vi "ClusterToArray_AssmeblyFeatures.vi"(11 "value":T1) -> (3 "Array":T2(array[cluster]))   [LabVIEW 2019]
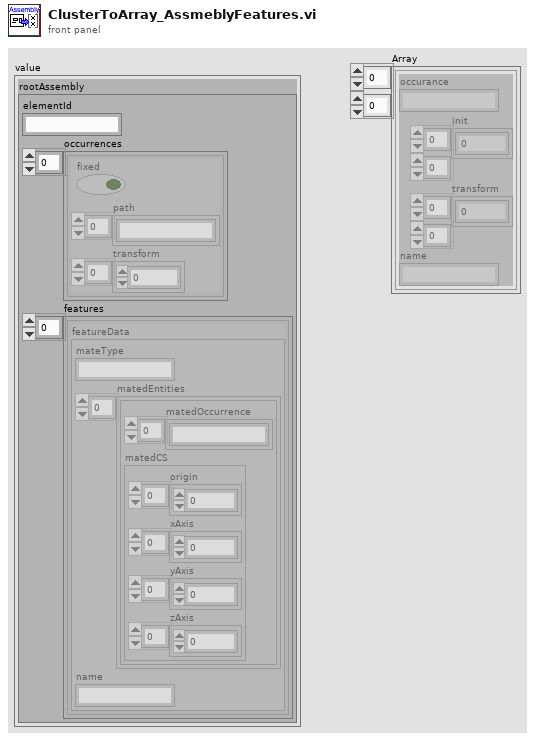
[diagram p1: front panel]
types:
  T1 = cluster{"rootAssembly":cluster{"elementId":string, "occurrences":cluster{"fixed":bool, "path":string[], "transform":dbl[]}[], "features":cluster{"featureData":cluster{"mateType":string, "matedEntities":cluster{"matedOccurrence":string[], "matedCS":cluster{"origin":dbl[], "xAxis":dbl[], "yAxis":dbl[], "zAxis":dbl[]}}[], "name":string}}[]}}
  T2 = cluster{"occurance":string, "init":dbl[][], "transform":dbl[][], "name":string}[][]
  T3 = cluster{"featureData":cluster{"mateType":string, "matedEntities":cluster{"matedOccurrence":string[], "matedCS":cluster{"origin":dbl[], "xAxis":dbl[], "yAxis":dbl[], "zAxis":dbl[]}}[], "name":string}}[]
  T4 = cluster{"fixed":bool, "path":string[], "transform":dbl[]}[]
  T5 = cluster{"occurance":string, "init":dbl[][], "transform":dbl[][], "name":string}
  T6 = cluster{"occurance":string, "init":dbl[][], "transform":dbl[][], "name":string}[]
  T7 = cluster{"matedOccurrence":string[], "matedCS":cluster{"origin":dbl[], "xAxis":dbl[], "yAxis":dbl[], "zAxis":dbl[]}}[]
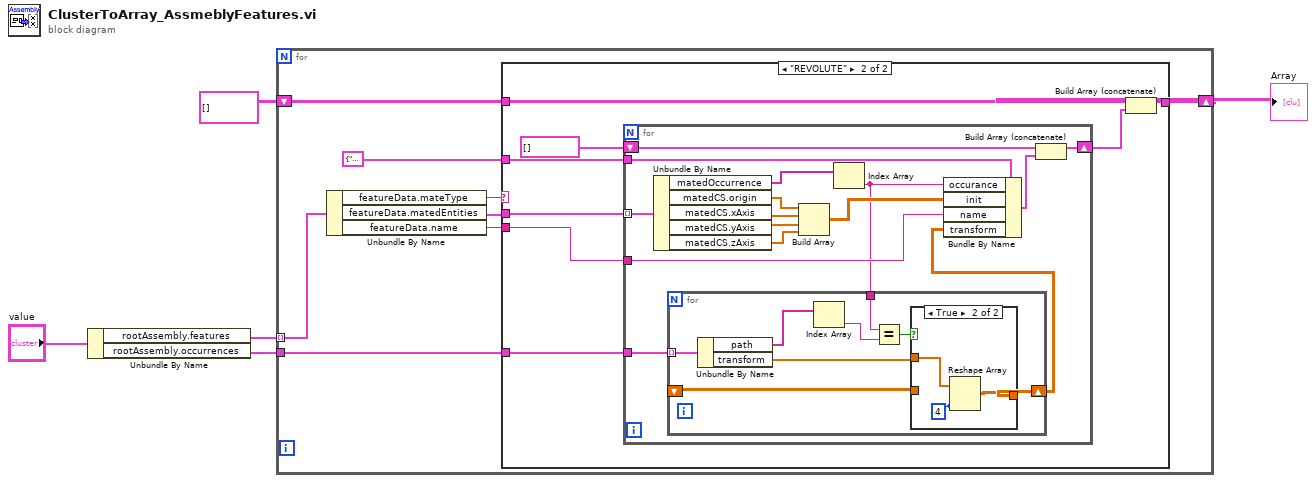
[diagram p0: block diagram]
diagram:
  n1 = Unbundle By Name("value") -> ("rootAssembly.features"=w2:T3, "rootAssembly.occurrences"=w5:T4)
  n2 = for {
    tunnel: w2 -> [w13] mode=indexing
    shift-right: [w7] -> w4
    shift-left: T2 [] -> [w8]
    tunnel: w5 -> [w6]
    n3 = Unbundle By Name(w13) -> ("featureData.mateType"=w12:string, "featureData.matedEntities"=w11:T7, "featureData.name"=w9:string)
    n4 = case shown="\"REVOLUTE\"" w12 {
      tunnel: w11 -> [_ w22]
      tunnel: T5 {"occurance"="", "init"=[], "transform"=[], "name"=""} -> [_ w21]
      tunnel: w9 -> [_ w15]
      tunnel: w8 -> [w14 w18]
      tunnel: [w14 w17] -> w7
      tunnel: w6 -> [_ w16]
      frame "False", Default {
      }
      frame "REVOLUTE" {
        n5 = for {
          tunnel: w22 -> [w37] mode=indexing
          tunnel: w21 -> [w36]
          shift-right: [w27] -> w19
          shift-left: T6 [] ("Array 2") -> [w26]
          tunnel: w15 -> [w29]
          tunnel: w16 -> [w25]
          n6 = Unbundle By Name(w37) -> ("matedOccurrence"=w35:string[], "matedCS.origin"=w34:dbl[], "matedCS.xAxis"=w33:dbl[], "matedCS.yAxis"=w32:dbl[], "matedCS.zAxis"=w31:dbl[])
          n7 = Build Array(w34, w33, w32, w31) -> (w30:dbl[][])
          n8 = Index Array(array=w35) -> (element=w24:string)  [unwired: 1 in]
          n9 = for {
            tunnel: w25 -> [w45] mode=indexing
            tunnel: w24 -> [w39]
            shift-right: [w41] -> w23
            shift-left: _ -> [w40]
            n10 = Unbundle By Name(w45) -> ("path"=w44:string[], "transform"=w42:dbl[])
            n11 = Index Array(array=w44) -> (element=w38:string)  [unwired: 1 in]
            n12 = Equal?(x=w39, y=w38) -> (x = y?=w43:bool)
            n13 = case shown="True" w43 {
              tunnel: w42 -> [_ w47]
              tunnel: [w46 w49] -> w41
              tunnel: w40 -> [w46 _]
              frame False {
              }
              frame True {
                w48 = 4 ("dimension size")
                n14 = Reshape Array(w47, w48, w48) -> (w49:dbl[][])
              }
            }
          }
          n15 = Bundle By Name(cluster=w36, "occurance"=w24, "init"=w30, "name"=w29, "transform"=w23) -> (w28:T5)
          n16 = Build Array (concatenate)(w26, w28) -> (w27:T6)
        }
        n17 = Build Array (concatenate)(w18, w19) -> (w17:T2)
      }
    }
  }
  "Array" <- w4
